vi "getAllLiteralsFromName.vi"(8 "error in (no error)":errorcluster, 10 "name":string, 11 "Enumeration in":refnum<class "Enumeration.lvclass">) -> (0 "error out":errorcluster, 1 "literals":string[](array[string]), 2 "name":string, 3 "Enumeration out":refnum<class "Enumeration.lvclass">)   [LabVIEW 2016, in "Enumeration.lvclass"]
uses:
  Enumeration.lvclass
  Enumeration.lvclass/Enumeration.ctl
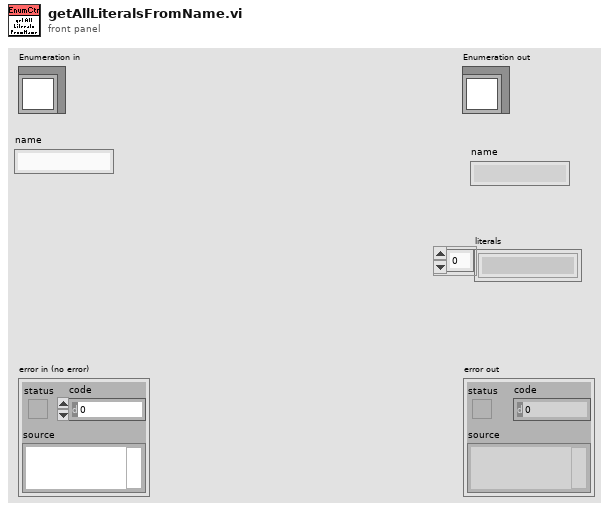
[diagram p1: front panel]
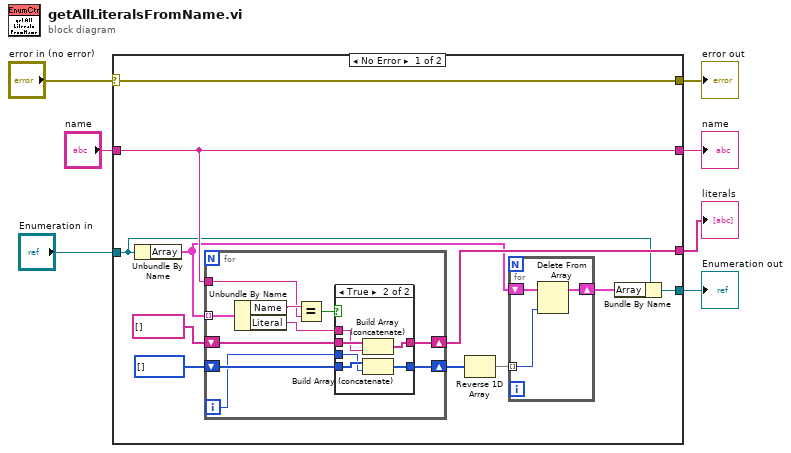
[diagram p0: block diagram]
diagram:
  n1 = case shown="No Error" "error in (no error)" {
    selector: "error in (no error)" -> [w18 w41]
    tunnel: [w18 w41] -> w6
    tunnel: [w11 w40] -> w4
    tunnel: "Enumeration in" -> [w12 w40]
    tunnel: "name" -> [w16 _]
    tunnel: [w16 _] -> w2
    tunnel: [w15 _] -> w1
    frame No Error {
      n2 = Unbundle By Name(w12) -> ("Array"=w8:cluster{"Name":string, "Literal":string}[])
      n3 = for {
        tunnel: w8 -> [w31] mode=indexing
        tunnel: w16 -> [w28]
        shift-right: [w25] -> w15
        shift-left: string[] [] -> [w27]
        shift-right: [w23] -> w10
        shift-left: i32[] [] -> [w24]
        i -> [w22]
        n4 = Unbundle By Name(w31) -> ("Name"=w29:string, "Literal"=w26:string)
        n5 = Equal?(x=w29, y=w28) -> (x = y?=w30:bool)
        n6 = case shown="True" w30 {
          tunnel: w27 -> [w33 w39]
          tunnel: w26 -> [_ w38]
          tunnel: [w33 w37] -> w25
          tunnel: w24 -> [w32 w36]
          tunnel: w22 -> [_ w35]
          tunnel: [w32 w34] -> w23
          frame False {
          }
          frame True {
            n7 = Build Array (concatenate)(w39, w38) -> (w37:string[])
            n8 = Build Array (concatenate)(w36, w35) -> (w34:i32[])
          }
        }
      }
      n9 = Reverse 1D Array(array=w10) -> (reversed array=w9:i32[])
      n10 = for {
        tunnel: w9 -> [w20] mode=indexing
        shift-right: [w21] -> w13
        shift-left: w8 -> [w19]
        n11 = Delete From Array(array=w19, index=w20) -> (array with subset deleted=w21:cluster{"Name":string, "Literal":string}[])  [unwired: 1 in, 1 out]
      }
      n12 = Bundle By Name(cluster=w12, "Array"=w13) -> (w11:refnum<class "Enumeration.lvclass">)
    }
    frame Error {
    }
  }
  "error out" <- w6
  "Enumeration out" <- w4
  "name" <- w2
  "literals" <- w1
